vi "Main.vi"(7 "error in (no error)":errorcluster, 10 "ModuleAdmin":refnum<class "ModuleAdmin.lvclass">) -> ()   [LabVIEW 2018, in "AcPwrPlugins.lvlib"]
doc: "This VI is the critical engine of the AcPwr Plugin. It makes all the initialize, configure, and etc calls to the instrument drivers using their specifica API functions based upon the loaded configuration file."
uses:
  AcPwrPlugins.lvlib
  <userlib>/NIST/ModuleAdminLib/ModuleAdmin/ModuleAdmin.lvclass
  C:/Program Files (x86)/National Instruments/LabVIEW 2018/user.lib/NIST/ModuleAdminLib/ModuleAdminBase/ModuleAdminBase.lvclass
  AcPwrBaseClass/AcPwrBase.lvclass
  C:/Program Files (x86)/National Instruments/LabVIEW 2018/user.lib/NIST/BaseClasses/BasePlugin_class/BasePlugin.lvclass
  AcPwrShared/clStopArgument.ctl
  <userlib>/NIST/ModuleAdminLib/ModuleAdmin/ModuleAdmin.lvclass/ModuleAdmin.ctl
  <userlib>/NIST/BaseClasses/BasePlugin_class/BasePlugin.lvclass/BasePlugin.ctl
  <vilib>/Utility/error.llb/DialogType.ctl
  <userlib>/NIST/ModuleAdminLib/ModuleAdmin/Accessors/Read ShowPanel_.vi
  <userlib>/NIST/ModuleAdminLib/ModuleAdmin/Accessors/Write ShowPanel_.vi
  <userlib>/NIST/BaseClasses/BasePlugin_class/Accessors/Write PluginIniFilePath.vi
  <userlib>/NIST/BaseClasses/BasePlugin_class/Accessors/Read PluginIniFilePath.vi
  <userlib>/NIST/ModuleAdminLib/ModuleAdmin/Accessors/Read CloneRegRef.vi
  <extravilib>/ChannelInstances/Tag-bool/Read With Abort.vi
  <extravilib>/ChannelInstances/Tag-bool/Write With Abort.vi
  <extravilib>/ChannelInstances/Tag-bool/Instantiate.vi
  <extravilib>/ChannelInstances/Tag-bool/EndpointRead.vi
  <vilib>/Utility/error.llb/Error Cluster From Error Code.vi
  <extravilib>/ChannelInstances/Tag-bool/Endpoint.vi
  <vilib>/ErrorRing/Error Ring.xnode
  <userlib>/NIST/ModuleAdminLib/CloneRegistration/CloneRegistration.lvclass
  AcPwrShared/AcPwrShared.lvlib
  <userlib>/NIST/BaseClasses/Object_class/BaseObject.lvclass
  <userlib>/NIST/ModuleAdminLib/ModuleAdmin.lvlib
  <extravilib>/ChannelInstances/Tag-bool.lvlib
panel:
  out "RunTime(ms)":u32
  out "error out":errorcluster
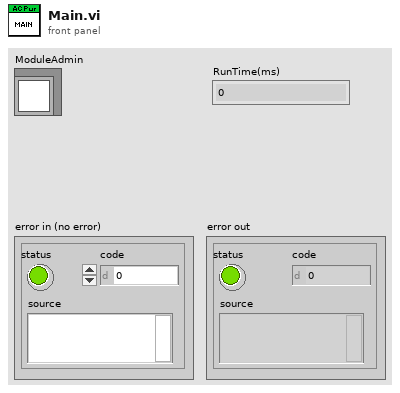
[diagram p1: front panel]
types:
  T1 = typedef "AcPwrShared.lvlib/clRequestEvents.ctl" = cluster{"StopRequest":refnum<user-event>, "PathToINI":refnum<user-event>, " LoadPlugin":refnum<user-event>, "ShowPanel":refnum<user-event>, "PrefDlg":refnum<user-event>, "InitAcPwr":refnum<user-event>, "Reset":refnum<user-event>, "Close":refnum<user-event>, "StopMeas":refnum<user-event>, "StartMeas":refnum<user-event>, "ConfigDevice":refnum<user-event>, "DeviceOn":refnum<user-event>, "DeviceOff":refnum<user-event>, "GetSettings":refnum<user-event>, "SetSettings":refnum<user-event>}
  T2 = typedef "AcPwrShared.lvlib/clBroadcastEvents.ctl" = cluster{"DidInit":refnum<user-event>, "StatusUpdate":refnum<user-event>, "ErrorReport":refnum<user-event>, "DidStop":refnum<user-event>, "PathToINI":refnum<user-event>, "Measurements":refnum<user-event>, "LoadConfigFile":refnum<user-event>, "GetSettings":refnum<user-event>, "SetSettings":refnum<user-event>, "GetType&ID":refnum<user-event>, "GotSettings":refnum<user-event>}
  T3 = typedef "AcPwrShared.lvlib/clStopArgument.ctl" = cluster{"Exit via Stop Module Req?":bool, "Wait for Module to stop?":bool, "ModuleAdmin":refnum<class "ModuleAdmin.lvclass">}
  T4 = enum32{"Invalid", "Standard", "Closed", "Hidden", "Minimized", "Maximized"}
  T5 = typedef "Tag-bool.lvlib/))Channel.ctl" = refnum<queue>
  T6 = typedef "DialogType.ctl" = u16
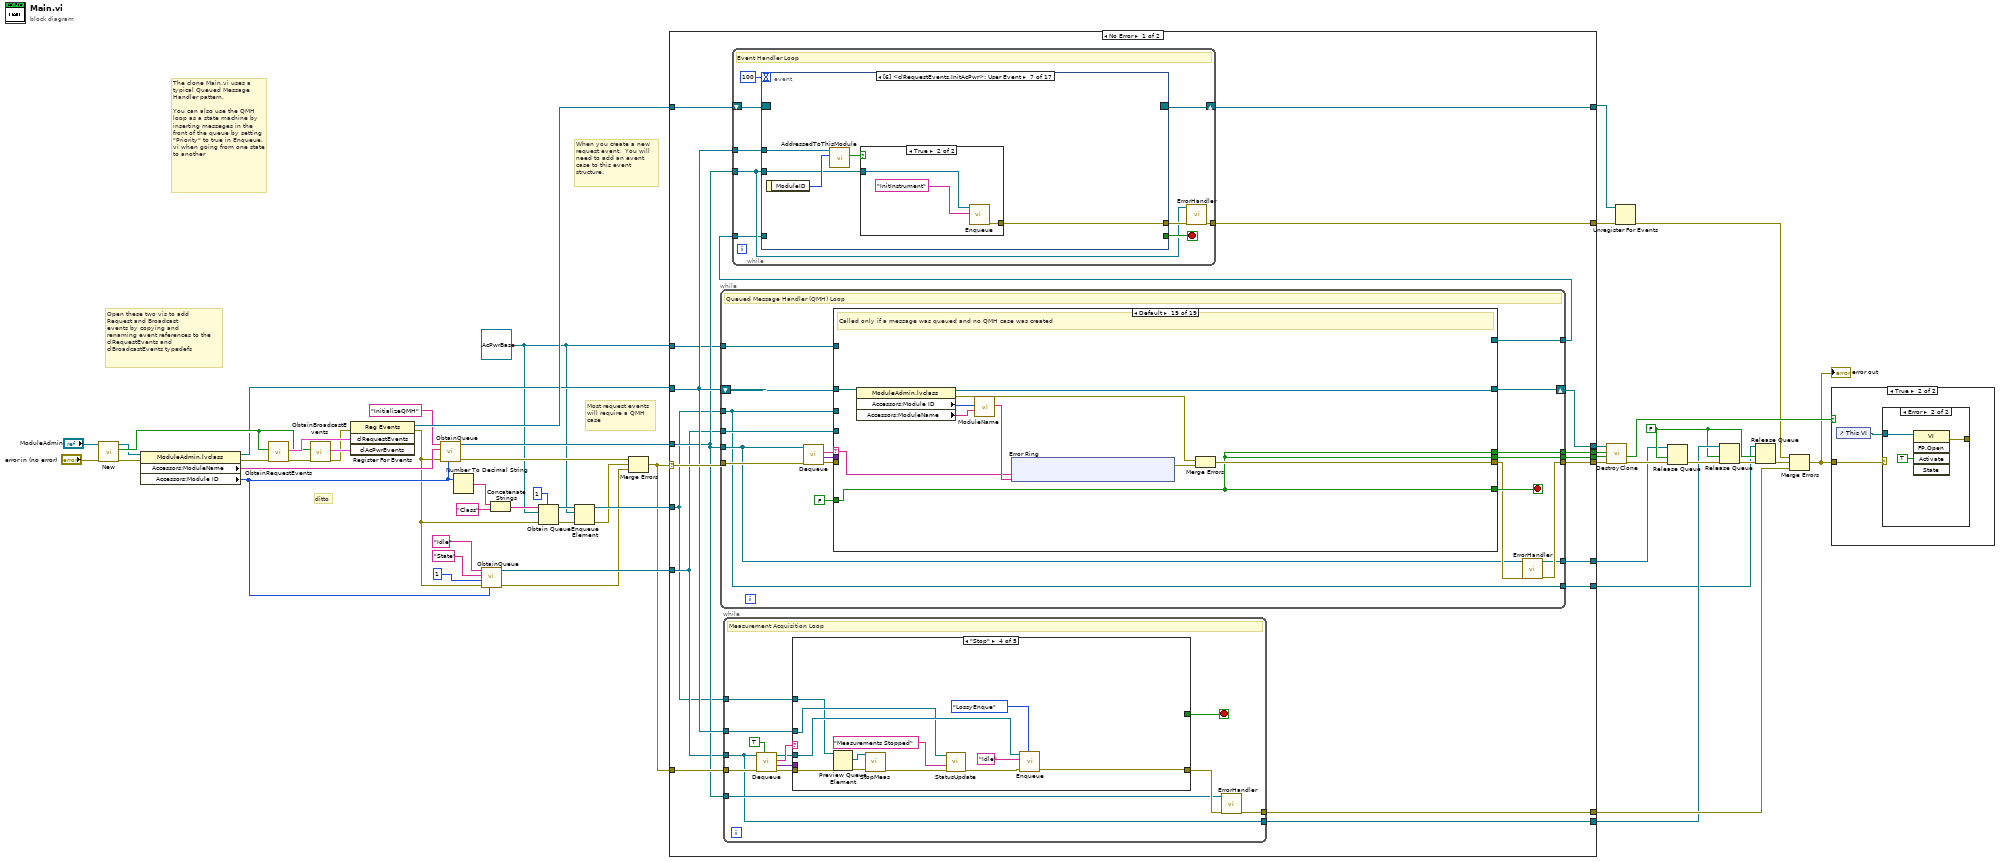
[diagram p0: block diagram]
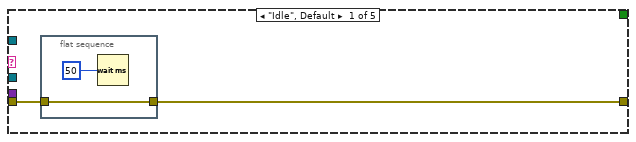
[diagram p2: hidden frame]
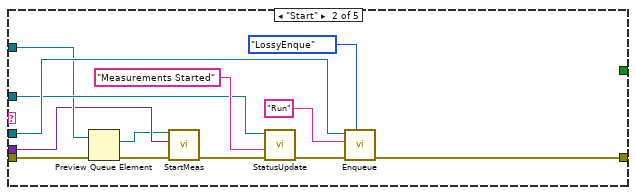
[diagram p3: hidden frame]
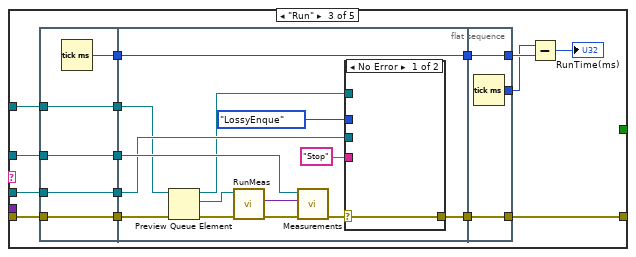
[diagram p4: hidden frame]
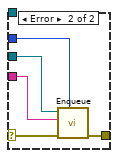
[diagram p5: hidden frame]
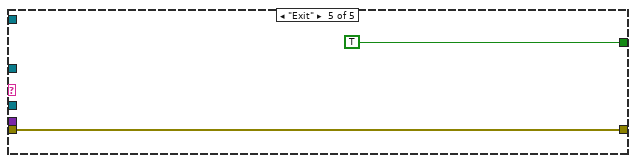
[diagram p6: hidden frame]
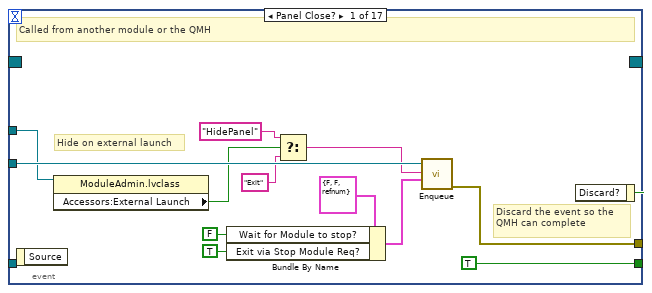
[diagram p7: hidden frame]
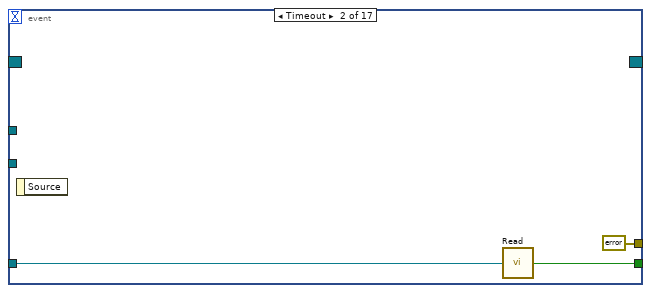
[diagram p8: hidden frame]
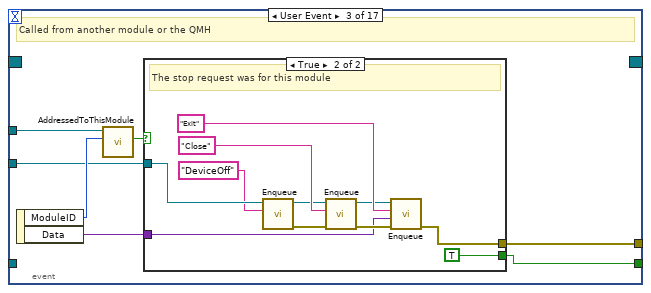
[diagram p9: hidden frame]
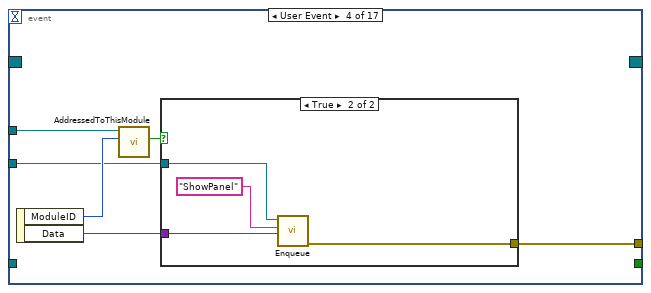
[diagram p11: hidden frame]
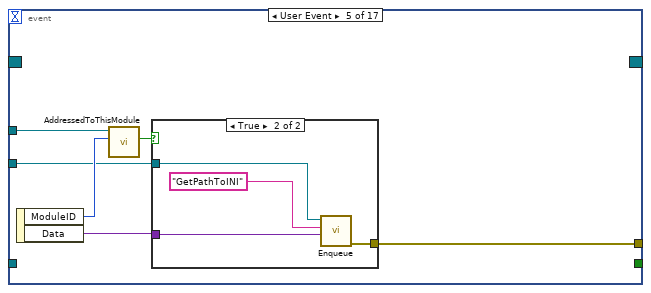
[diagram p13: hidden frame]
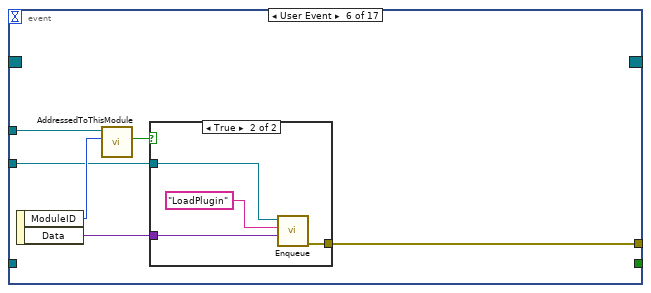
[diagram p15: hidden frame]
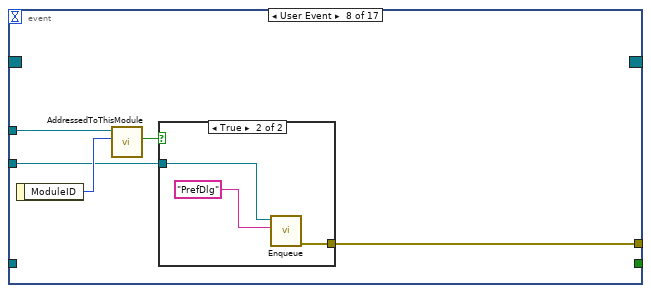
[diagram p18: hidden frame]
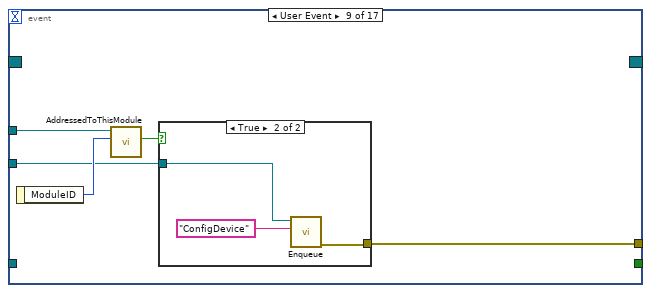
[diagram p20: hidden frame]
diagram:
  w2 = refnum<class "AcPwrBase.lvclass"> refnum ("MyPlugins.lvlib:MyPluginsBase.lvclass")
  w20 = FALSE ("force destroy? (F)")
  # "The clone Main.vi uses a typical Queued Message Handler pattern.  \n\nYou can also use the QMH loop as a state machine by inserting messeges in the front of the queue by setting \"Priority\" to true in Enqueue.vi when going from one state to another"
  # "Open these two vis to add\nRequest and Broadcast \nevents by copying and \nrenaming event references to the \nclRequestEvents and \nclBroadcastEvents typedefs"
  # "ditto"
  # "Most request events\nwill require a QMH\ncase"
  # "When you create a new request event.  You will need to add an event case to this event structure."
  n1 = call <userlib>:"New.vi"("error in (no error)"="error in (no error)", "ModuleAdmin"="ModuleAdmin") -> ("error out"=w34:errorcluster, "First?"=w47:bool, "ModuleAdmin"=w35:refnum<class "ModuleAdmin.lvclass">)  [unwired: 6 in, 1 out]
  n2 = property class="ModuleAdmin.lvclass"(reference=w35, error in=w34) -> (reference out=w31:refnum<class "ModuleAdmin.lvclass">, error out=w33:errorcluster, "Accessors:ModuleName"=w32:string, "Accessors:Module ID"=w24:i32)
  n3 = call "ObtainRequestEvents.vi"("error in (no error)"=w33, "CreateNew (F)"=w47) -> ("error out"=w46:errorcluster, "clRequestEvents"=w49:T1)  [unwired: 8 in]
  n4 = call "ObtainBroadcastEvents.vi"("error in (no error)"=w46, "CreateNew? (F)"=w47) -> ("error out"=w14:errorcluster, "clAcPwrEvents"=w45:T2)  [unwired: 8 in]
  n5 = register-events(error in=w14, w49, w45) -> (reference out=w44:refnum<event-registration>, error out=w13:errorcluster)  [unwired: 1 in]
  n6 = call "ObtainQueue.vi"("ModuleID"=w24, "error in (no error)"=w13, "ModuleName"=w32, "Initial Message"="InitializeQMH" ("ModuleName")) -> ("error out"=w9:errorcluster, "MessageQueue"=w48:refnum<queue>)  [unwired: 6 in]
  n7 = Number To Decimal String(number=w24) -> (decimal integer string=w25:string)  [unwired: 1 in]
  n8 = call "ObtainQueue.vi"("ModuleID"=w24, "error in (no error)"=w13, "max queue size (-1, unlimited)"=1, "ModuleName"="State", "Initial Message"="Idle") -> ("error out"=w7:errorcluster, "MessageQueue"=w29:refnum<queue>)  [unwired: 5 in]
  n9 = Concatenate Strings(w25, "Class" ("ModuleName")) -> (w22:string)
  n10 = Obtain Queue(max queue size (-1, unlimited)=1, name (unnamed)=w22, element data type=w2, error in (no error)=w13) -> (queue out=w16:refnum<queue>, error out=w21:errorcluster)  [unwired: 1 in, 1 out]
  n11 = Enqueue Element(queue=w16, element=w2, error in (no error)=w21) -> (queue out=w15:refnum<queue>, error out=w8:errorcluster)  [unwired: 1 in, 1 out]
  n12 = Merge Errors(w9, w8, w7) -> (w6:errorcluster)
  n13 = case shown="No Error" w6 {
    selector: w6 -> [w70 w982]
    tunnel: w48 -> [w59 w971]
    tunnel: w31 -> [w60 w980]
    tunnel: [w69 w972] -> w3
    tunnel: w44 -> [w68 w976]
    tunnel: [w67 w979] -> w4
    tunnel: [w66 _] -> w42
    tunnel: [w65 _] -> w41
    tunnel: [w64 w972] -> w39
    tunnel: [w63 w976] -> w38
    tunnel: w6 -> [w62 w975]
    tunnel: [w61 w975] -> w30
    tunnel: w29 -> [w57 w974]
    tunnel: [w58 w974] -> w27
    tunnel: w15 -> [w56 w973]
    tunnel: [w55 w973] -> w17
    tunnel: w2 -> [w53 _]
    tunnel: [w52 w971] -> w1
    frame No Error {
      n14 = while {
        tunnel: w59 -> [w343]
        tunnel: w70 -> [w352]
        tunnel: [w342] -> w69
        tunnel: [w347] -> w66
        tunnel: [w346] -> w65
        shift-right: [w344] -> w67
        shift-left: w60 -> [w348]
        tunnel: w57 -> [w341]
        tunnel: w56 -> [w340]
        tunnel: [w340] -> w55
        tunnel: [w339] -> w54
        tunnel: w53 -> [w338]
        tunnel: [w337] -> w52
        stop <- w353 stop-if-true
        # "Queued Message Handler (QMH) Loop"
        n15 = call "Dequeue.vi"("error in (no error)"=w352, "MessageQueue"=w343) -> ("error out"=w351:errorcluster, "Message Data"=w349:variant, "Message"=w350:string)  [unwired: 5 in, 2 out]
        n16 = case shown="Default" w350 {
          selector: w350 -> [_ _ _ _ _ _ _ _ _ _ _ _ _ _ _ _ _ _ w959]
          tunnel: [w354 w385 w398 w446 w458 w489 w542 w595 w608 w664 w714 w765 w773 w780 w870 w893 w917 w930 w953] -> w353
          tunnel: w348 -> [w376 w394 w403 w455 w469 w501 w554 w597 w621 w673 w722 w770 w777 w788 w885 w909 w920 w935 w962]
          tunnel: [w365 w388 w404 w456 w468 w500 w553 w603 w620 w675 w725 w771 w778 w789 w887 w910 w928 w936 w954] -> w345
          tunnel: w351 -> [w358 w397 w413 w450 w465 w499 w552 w607 w619 w671 w721 w772 w779 w784 w874 w897 w924 w933 _]
          tunnel: w349 -> [_ w396 w415 _ _ _ _ w596 w609 _ _ w766 _ _ _ _ w921 w943 _]
          tunnel: [w354 w385 w398 w446 w458 w489 w542 w595 w608 w664 w714 w765 w773 w780 w870 w893 w926 w929 w953] -> w347
          tunnel: [w354 w385 w398 w446 w458 w489 w542 w595 w608 w664 w714 w765 w773 w780 w870 w893 w925 w929 w953] -> w346
          tunnel: [w359 w393 w401 w454 w467 w496 w549 w601 w616 w672 w723 w770 w777 w787 w884 w908 w920 w934 w957] -> w344
          tunnel: w341 -> [_ _ _ _ w463 w495 w548 _ w615 w674 w724 w769 w776 w785 w872 w900 w922 _ _]
          tunnel: w340 -> [_ _ w400 w448 w462 w498 w551 w606 w618 w670 w720 _ _ w781 w875 w895 _ _ _]
          tunnel: [_ _ _ _ _ _ _ _ _ _ _ _ _ _ _ _ w916 w932 _] -> w339
          tunnel: w338 -> [_ _ w399 _ _ _ _ _ _ _ _ _ _ _ _ _ _ _ _]
          tunnel: FALSE ("Error/Exit") -> [w354 w385 w398 w446 w458 w489 w542 w595 w608 w664 w714 w765 w773 w780 w870 w893 _ w929 w953]
          frame "InitializeQMH" {
            # "After the QMH, Class, and State Queue have been created this loop enters the intialize phase."
            n17 = property class="ModuleAdmin.lvclass"(reference=w376, error in=w358) -> (reference out=w363:refnum<class "ModuleAdmin.lvclass">, error out=w373:errorcluster, "Accessors:ShowPanel_"=w362:bool, "Accessors:External Launch"=w361:bool, "Accessors:Module ID"=w356:i32, "Accessors:ModuleName"=w357:string)
            n18 = Compound Arithmetic op=OR(w362, invert w361) -> (w360:bool)
            n19 = Select(t=T4."Standard" ("Front Panel Window:State"), s=w360, f=T4."Hidden" ("Front Panel Window:State")) -> (s? t:f=w369:T4)
            n20 = invoke class="VI" method="FP.Open"(error in=w373, "State"=w369) -> (reference out=w355:refnum<vi>, error out=w372:errorcluster)  [unwired: 3 in, 3 out]
            n21 = call <userlib>:"ModuleName.vi"("Name"=w357, "ModuleID"=w356) -> ("ModuleName"=w368:string)  [unwired: 9 in]
            n22 = property class="VI"(reference=w355, error in=w372, "Front Panel.Title"=w368) -> (reference out=w375:refnum<vi>, error out=w374:errorcluster)
            n23 = invoke class="VI" method="FP.Center"(reference=w375, error in=w374) -> (error out=w364:errorcluster)  [unwired: 1 in, 2 out]
            n24 = case shown="True" w361 {
              tunnel: [w377 w383] -> w366
              tunnel: [w378 w380] -> w359
              tunnel: w364 -> [w377 w382]
              tunnel: w363 -> [w378 w379]
              frame False {
              }
              frame True {
                n25 = call <userlib>:"WaitOnModuleSync.vi"("error in (no error)"=w382, "ModuleAdmin"=w379) -> ("error out"=w384:errorcluster, "ModuleAdmin"=w381:refnum<class "ModuleAdmin.lvclass">)  [unwired: 8 in]
                n26 = call <userlib>:"WaitOnEventSync.vi"("error in (no error)"=w384, "ModuleAdmin"=w381) -> ("error out"=w383:errorcluster, "ModuleAdmin"=w380:refnum<class "ModuleAdmin.lvclass">)  [unwired: 8 in]
              }
            }
            n27 = call "DidInit.vi"("Init?"=TRUE, "error in (no error)"=w366, "ModuleAdmin"=w359) -> ("error out"=w365:errorcluster)  [unwired: 8 in]
          }
          frame "ShowPanel" {
            # "The front panel can be shown or hidden"
            n28 = Variant To Data(error in=w397, type=TRUE, Variant=w396) -> (data=w390:bool, error out=w387:errorcluster)
            n29 = property class="ModuleAdmin.lvclass"(reference=w394, error in=w387, "Accessors:ShowPanel_"=w390) -> (reference out=w393:refnum<class "ModuleAdmin.lvclass">, error out=w386:errorcluster)
            n30 = Select(t=T4."Standard" ("Front Panel Window:State"), s=w390, f=T4."Hidden" ("Front Panel Window:State")) -> (s? t:f=w389:T4)
            n31 = property class="VI"(error in=w386, "FP.State"=w389) -> (error out=w388:errorcluster)  [unwired: 1 in, 1 out]
          }
          frame "LoadPlugin" {
            # "Dynamically loads and initializes a plugin from the .ini file"
            n32 = Variant To Data(error in=w413, type=path "", Variant=w415) -> (data=w402:path, error out=w412:errorcluster)
            n33 = Current VI's Path() -> (path=w410:path)
            n34 = call <userlib>:"GetPathToClass.vi"("error in (no error)"=w412, "configuration file path"=w402) -> ("error IO"=w408:errorcluster, "PathToClass"=w411:path)  [unwired: 8 in]
            n35 = Build Path(base path=w410, name or relative path=w411) -> (appended path=w409:path)
            n36 = call <vilib>:"Check if File or Folder Exists.vi"("error in (no error)"=w408, "path"=w409) -> ("error out"=w405:errorcluster, "file or folder exists?"=w407:bool, "dup path"=w406:path)  [unwired: 7 in]
            n37 = case shown="True" w407 {
              tunnel: w406 -> [w418 w428]
              tunnel: w405 -> [_ w433]
              tunnel: [w417 w443] -> w404
              tunnel: w403 -> [w416 w439]
              tunnel: w402 -> [_ w440]
              tunnel: [w416 w438] -> w401
              tunnel: w400 -> [_ w432]
              tunnel: w399 -> [_ w427]
              frame False {
                n38 = Path To String(path=w418) -> (string=w419:string)
                n39 = xnode "Error Ring"("parameter 0"=w419) -> ("error out"=w417:errorcluster)
              }
              frame True {
                n40 = Strip Path(path=w428) -> (name=w431:string)  [unwired: 1 out]
                n41 = call-dynamic "LoadClassFromFile.vi"("error in (no error)"=w433, "class path"=w428, "reference in"=w427) -> ("error out"=w441:errorcluster, "reference out"=w442:refnum<class "AcPwrBase.lvclass">)  [unwired: 7 in]
                n42 = property class="AcPwrBase.lvclass"(reference=w442, error in=w441, "Accessors:PluginIniFilePath"=w440) -> (reference out=w437:refnum<class "AcPwrBase.lvclass">, error out=w436:errorcluster)
                n43 = call-dynamic "DefaultFromIni.vi"("error in (no error)"=w436, "AcPwrBase"=w437) -> ("error out"=w434:errorcluster, "AcPwrBase"=w435:refnum<class "AcPwrBase.lvclass">)  [unwired: 8 in]
                n44 = Lossy Enqueue Element(queue=w432, element=w435, error in (no error)=w434) -> (error out=w429:errorcluster)  [unwired: 3 out]
                n45 = Format Into String(format string="Plugin %s loaded ", error in=w429, w431) -> (resulting string=w444:string, error out=w430:errorcluster)  [unwired: 1 in]
                n46 = call "StatusUpdate.vi"("error in (no error)"=w430, "Status"=w444, "Module"=w439) -> ("error out"=w443:errorcluster, "Module"=w438:refnum<class "ModuleAdmin.lvclass">)  [unwired: 7 in]
              }
            }
          }
          frame "GetPathToINI" {
            # "Broadcast the path to the .ini file"
            n47 = Preview Queue Element(queue=w448, error in (no error)=w450) -> (element=w453:refnum<class "AcPwrBase.lvclass">, error out=w449:errorcluster)  [unwired: 1 in, 2 out]
            n48 = property class="AcPwrBase.lvclass"(reference=w453, error in=w449) -> (error out=w452:errorcluster, "Accessors:PluginIniFilePath"=w447:path)  [unwired: 1 out]
            n49 = property class="ModuleAdmin.lvclass"(reference=w455, error in=w452) -> (reference out=w454:refnum<class "ModuleAdmin.lvclass">, error out=w451:errorcluster, "Accessors:Module ID"=w457:i32)
            n50 = call "PathToINI.vi"("error in (no error)"=w451, "PathToINI"=w447, "ModuleID"=w457) -> ("error out"=w456:errorcluster)  [unwired: 8 in]
          }
          frame "InitInstrument" {
            n51 = call "Dequeue.vi"("PreviewQueue(F)"=TRUE, "error in (no error)"=w465, "MessageQueue"=w463) -> ("error out"=w464:errorcluster, "Message"=w460:string)  [unwired: 4 in, 3 out]
            n52 = Equal?(x="Run" ("y"), y=w460) -> (x = y?=w466:bool)
            n53 = case shown="False" w466 {
              tunnel: w469 -> [w481 w483]
              tunnel: [w480 w482] -> w468
              tunnel: [w478 w483] -> w467
              tunnel: w464 -> [w475 _]
              tunnel: w462 -> [w473 _]
              frame False {
                n54 = Preview Queue Element(queue=w473, error in (no error)=w475) -> (queue out=w471:refnum<queue>, element=w477:refnum<class "AcPwrBase.lvclass">, error out=w474:errorcluster)  [unwired: 1 in, 1 out]
                n55 = call-dynamic "Initialize.vi"("error in (no error)"=w474, "AcPwrBase in"=w477) -> ("error out"=w472:errorcluster, "AcPwrBase out"=w476:refnum<class "AcPwrBase.lvclass">)  [unwired: 8 in]
                n56 = Lossy Enqueue Element(queue=w471, element=w476, error in (no error)=w472) -> (error out=w470:errorcluster)  [unwired: 3 out]
                n57 = call "StatusUpdate.vi"("error in (no error)"=w470, "Status"="Device Initialized", "Module"=w481) -> ("error out"=w480:errorcluster, "Module"=w478:refnum<class "ModuleAdmin.lvclass">)  [unwired: 7 in]
              }
              frame True {
                n58 = xnode "Error Ring"() -> ("error out"=w482:errorcluster)
              }
            }
          }
          frame "ConfigDevice" {
            n59 = Preview Queue Element(queue=w498, error in (no error)=w499) -> (queue out=w497:refnum<queue>, element=w493:refnum<class "AcPwrBase.lvclass">, error out=w494:errorcluster)  [unwired: 1 in, 1 out]
            n60 = call-dynamic "ChangeWhileMeasuring.vi"("error in (no error)"=w494, "AcPwrBase in"=w493) -> ("error out"=w492:errorcluster, "OutputOrLoadValue"=w490:bool, "AcPwrBase out"=w491:refnum<class "AcPwrBase.lvclass">)  [unwired: 6 in, 1 out]
            n61 = case shown="False" w490 {
              tunnel: w501 -> [w511 w536]
              tunnel: w491 -> [w509 w518]
              tunnel: [w508 w528] -> w500
              tunnel: w492 -> [w507 w521]
              tunnel: w497 -> [w503 w525]
              tunnel: [w506 w524] -> w496
              tunnel: w495 -> [_ w520]
              frame True {
                n62 = call-dynamic "ConfigDevice.vi"("error in (no error)"=w507, "AcPwrBase in"=w509) -> ("error out"=w505:errorcluster, "AcPwrBase out"=w502:refnum<class "AcPwrBase.lvclass">)  [unwired: 8 in]
                n63 = Lossy Enqueue Element(queue=w503, element=w502, error in (no error)=w505) -> (error out=w504:errorcluster)  [unwired: 3 out]
                n64 = call "StatusUpdate.vi"("error in (no error)"=w504, "Status"="Device Configured", "Module"=w511) -> ("error out"=w508:errorcluster, "Module"=w506:refnum<class "ModuleAdmin.lvclass">)  [unwired: 7 in]
              }
              frame False {
                w533 = TRUE ("OverwriteClass? (F)")
                n65 = call "Dequeue.vi"("PreviewQueue(F)"=TRUE, "error in (no error)"=w521, "MessageQueue"=w520) -> ("error out"=w519:errorcluster, "Message"=w513:string, "MessageQueue"=w512:refnum<queue>)  [unwired: 4 in, 2 out]
                n66 = Equal?(x="Run" ("y"), y=w513) -> (x = y?=w516:bool)
                n67 = call "CheckonIdle.vi"("MessageQueue"=w512, "OverwriteClass? (F)"=w533, "error in (no error)"=w519, "ChangeOccured? (F)"=w533, "AcPwrBase in"=w518) -> ("Error Out"=w534:errorcluster, "Write?"=w530:bool, "AcPwrBase out"=w532:refnum<class "AcPwrBase.lvclass">)  [unwired: 4 in]
                n68 = call-dynamic "ConfigDevice.vi"("error in (no error)"=w534, "AcPwrBase in"=w532) -> ("error out"=w527:errorcluster, "AcPwrBase out"=w531:refnum<class "AcPwrBase.lvclass">)  [unwired: 8 in]
                n69 = case shown="True" w530 {
                  tunnel: [w537 w541] -> w526
                  tunnel: w527 -> [w537 w540]
                  tunnel: w525 -> [_ w539]
                  tunnel: w531 -> [_ w538]
                  frame False {
                  }
                  frame True {
                    n70 = Lossy Enqueue Element(queue=w539, element=w538, error in (no error)=w540) -> (error out=w541:errorcluster)  [unwired: 3 out]
                  }
                }
                n71 = call "StatusUpdate.vi"("error in (no error)"=w526, "Status"="Device Configured", "Module"=w536) -> ("error out"=w529:errorcluster, "Module"=w524:refnum<class "ModuleAdmin.lvclass">)  [unwired: 7 in]
                n72 = Select(t="Start" ("strngStateIn"), s=w516, f=w513) -> (s? t:f=w514:string)
                n73 = call "Enqueue.vi"("EnqueType (Enque)"=enum16{"LossyEnque", "EnqueAtFront", "Enque"}."LossyEnque" ("Enum"), "error in (no error)"=w529, "Message"=w514, "MessageQueue"=w512) -> ("error out"=w528:errorcluster)  [unwired: 6 in, 1 out]
              }
            }
          }
          frame "ConfigPhases" {
            # "Need to reealy look into if this case is needed"
            n74 = Preview Queue Element(queue=w551, error in (no error)=w552) -> (queue out=w550:refnum<queue>, element=w546:refnum<class "AcPwrBase.lvclass">, error out=w547:errorcluster)  [unwired: 1 in, 1 out]
            n75 = call-dynamic "ChangeWhileMeasuring.vi"("error in (no error)"=w547, "AcPwrBase in"=w546) -> ("error out"=w545:errorcluster, "OutputOrLoadValue"=w543:bool, "AcPwrBase out"=w544:refnum<class "AcPwrBase.lvclass">)  [unwired: 6 in, 1 out]
            n76 = case shown="False" w543 {
              tunnel: w554 -> [w564 w589]
              tunnel: w544 -> [w557 w575]
              tunnel: [w562 w584] -> w553
              tunnel: w545 -> [w558 w578]
              tunnel: w550 -> [w559 w582]
              tunnel: [w561 w581] -> w549
              tunnel: w548 -> [_ w577]
              frame True {
                n77 = call-dynamic "ConfigPhases.vi"("error in (no error)"=w558, "AcPwrBase in"=w557) -> ("error out"=w556:errorcluster, "AcPwrBase out"=w555:refnum<class "AcPwrBase.lvclass">)  [unwired: 8 in]
                n78 = Lossy Enqueue Element(queue=w559, element=w555, error in (no error)=w556) -> (error out=w560:errorcluster)  [unwired: 3 out]
                n79 = call "StatusUpdate.vi"("error in (no error)"=w560, "Status"="PhaseAngle Configured", "Module"=w564) -> ("error out"=w562:errorcluster, "Module"=w561:refnum<class "ModuleAdmin.lvclass">)  [unwired: 7 in]
              }
              frame False {
                w587 = TRUE ("OverwriteClass? (F)")
                n80 = call "Dequeue.vi"("PreviewQueue(F)"=TRUE, "error in (no error)"=w578, "MessageQueue"=w577) -> ("error out"=w576:errorcluster, "Message"=w570:string, "MessageQueue"=w569:refnum<queue>)  [unwired: 4 in, 2 out]
                n81 = Equal?(x="Run" ("y"), y=w570) -> (x = y?=w573:bool)
                n82 = call "CheckonIdle.vi"("MessageQueue"=w569, "OverwriteClass? (F)"=w587, "error in (no error)"=w576, "ChangeOccured? (F)"=w587, "AcPwrBase in"=w575) -> ("Error Out"=w566:errorcluster, "Write?"=w586:bool, "AcPwrBase out"=w565:refnum<class "AcPwrBase.lvclass">)  [unwired: 4 in]
                n83 = call-dynamic "ConfigPhases.vi"("error in (no error)"=w566, "AcPwrBase in"=w565) -> ("error out"=w568:errorcluster, "AcPwrBase out"=w567:refnum<class "AcPwrBase.lvclass">)  [unwired: 8 in]
                n84 = case shown="True" w586 {
                  tunnel: [w590 w594] -> w583
                  tunnel: w568 -> [w590 w593]
                  tunnel: w582 -> [_ w592]
                  tunnel: w567 -> [_ w591]
                  frame False {
                  }
                  frame True {
                    n85 = Lossy Enqueue Element(queue=w592, element=w591, error in (no error)=w593) -> (error out=w594:errorcluster)  [unwired: 3 out]
                  }
                }
                n86 = call "StatusUpdate.vi"("error in (no error)"=w583, "Status"="PhaseAngle Configured", "Module"=w589) -> ("error out"=w585:errorcluster, "Module"=w581:refnum<class "ModuleAdmin.lvclass">)  [unwired: 7 in]
                n87 = Select(t="Start" ("strngStateIn"), s=w573, f=w570) -> (s? t:f=w571:string)
                n88 = call "Enqueue.vi"("EnqueType (Enque)"=enum16{"LossyEnque", "EnqueAtFront", "Enque"}."LossyEnque" ("Enum"), "error in (no error)"=w585, "Message"=w571, "MessageQueue"=w569) -> ("error out"=w584:errorcluster)  [unwired: 6 in, 1 out]
              }
            }
          }
          frame "GetSettings" {
            n89 = Preview Queue Element(queue=w606, error in (no error)=w607) -> (element=w604:refnum<class "AcPwrBase.lvclass">, error out=w605:errorcluster)  [unwired: 1 in, 2 out]
            n90 = call-dynamic "GetSettings.vi"("error in (no error)"=w605, "SettingsToRetrieve"=w596, "AcPwrBase in"=w604) -> ("error out"=w600:errorcluster, "RetrievedSettings"=w598:variant)  [unwired: 6 in, 1 out]
            n91 = call "Settings.vi"("error in (no error)"=w600, "variant"=w598, "Module"=w597) -> ("error out"=w599:errorcluster)  [unwired: 8 in]
            n92 = call "StatusUpdate.vi"("error in (no error)"=w599, "Status"="Settings Retrieved", "Module"=w597) -> ("error out"=w603:errorcluster, "Module"=w601:refnum<class "ModuleAdmin.lvclass">)  [unwired: 7 in]
          }
          frame "SetSettings" {
            n93 = Preview Queue Element(queue=w618, error in (no error)=w619) -> (queue out=w617:refnum<queue>, element=w613:refnum<class "AcPwrBase.lvclass">, error out=w614:errorcluster)  [unwired: 1 in, 1 out]
            n94 = call-dynamic "ChangeWhileMeasuring.vi"("error in (no error)"=w614, "AcPwrBase in"=w613) -> ("error out"=w612:errorcluster, "OutputOrLoadValue"=w610:bool, "AcPwrBase out"=w611:refnum<class "AcPwrBase.lvclass">)  [unwired: 6 in, 1 out]
            n95 = case shown="False" w610 {
              tunnel: w621 -> [w632 w658]
              tunnel: w611 -> [w625 w635]
              tunnel: [w630 w653] -> w620
              tunnel: w612 -> [w626 w647]
              tunnel: w617 -> [w627 w651]
              tunnel: [w629 w650] -> w616
              tunnel: w615 -> [_ w646]
              tunnel: w609 -> [w624 w636]
              frame True {
                n96 = call-dynamic "SetSettings.vi"("error in (no error)"=w626, "Variant"=w624, "AcPwrBase in"=w625) -> ("error out"=w622:errorcluster, "AcPwrBase Out"=w623:refnum<class "AcPwrBase.lvclass">)  [unwired: 7 in]
                n97 = Lossy Enqueue Element(queue=w627, element=w623, error in (no error)=w622) -> (error out=w628:errorcluster)  [unwired: 3 out]
                n98 = call "StatusUpdate.vi"("error in (no error)"=w628, "Status"="Settings Set", "Module"=w632) -> ("error out"=w630:errorcluster, "Module"=w629:refnum<class "ModuleAdmin.lvclass">)  [unwired: 7 in]
              }
              frame False {
                w656 = TRUE ("OverwriteClass? (F)")
                n99 = call "Dequeue.vi"("PreviewQueue(F)"=TRUE, "error in (no error)"=w647, "MessageQueue"=w646) -> ("error out"=w645:errorcluster, "Message"=w640:string, "MessageQueue"=w639:refnum<queue>)  [unwired: 4 in, 2 out]
                n100 = Equal?(x="Run" ("y"), y=w640) -> (x = y?=w643:bool)
                n101 = call "CheckonIdle.vi"("MessageQueue"=w639, "OverwriteClass? (F)"=w656, "error in (no error)"=w645, "ChangeOccured? (F)"=w656, "AcPwrBase in"=w635) -> ("Error Out"=w637:errorcluster, "Write?"=w655:bool, "AcPwrBase out"=w638:refnum<class "AcPwrBase.lvclass">)  [unwired: 4 in]
                n102 = call-dynamic "SetSettings.vi"("error in (no error)"=w637, "Variant"=w636, "AcPwrBase in"=w638) -> ("error out"=w633:errorcluster, "AcPwrBase Out"=w634:refnum<class "AcPwrBase.lvclass">)  [unwired: 7 in]
                n103 = Select(t="Start" ("strngStateIn"), s=w643, f=w640) -> (s? t:f=w641:string)
                n104 = case shown="True" w655 {
                  tunnel: [w659 w663] -> w652
                  tunnel: w633 -> [w659 w662]
                  tunnel: w651 -> [_ w661]
                  tunnel: w634 -> [_ w660]
                  frame False {
                  }
                  frame True {
                    n105 = Lossy Enqueue Element(queue=w661, element=w660, error in (no error)=w662) -> (error out=w663:errorcluster)  [unwired: 3 out]
                  }
                }
                n106 = call "StatusUpdate.vi"("error in (no error)"=w652, "Status"="Settings Set", "Module"=w658) -> ("error out"=w654:errorcluster, "Module"=w650:refnum<class "ModuleAdmin.lvclass">)  [unwired: 7 in]
                n107 = call "Enqueue.vi"("EnqueType (Enque)"=enum16{"LossyEnque", "EnqueAtFront", "Enque"}."LossyEnque" ("Enum"), "error in (no error)"=w654, "Message"=w641, "MessageQueue"=w639) -> ("error out"=w653:errorcluster)  [unwired: 6 in, 1 out]
              }
            }
          }
          frame "DeviceOn" {
            # "Turns the device on."
            n108 = Preview Queue Element(queue=w670, error in (no error)=w671) -> (element=w668:refnum<class "AcPwrBase.lvclass">, error out=w669:errorcluster)  [unwired: 1 in, 2 out]
            n109 = call-dynamic "ChangeWhileMeasuring.vi"("error in (no error)"=w669, "AcPwrBase in"=w668) -> ("error out"=w667:errorcluster, "OutputOrLoadValue"=w666:bool, "AcPwrBase out"=w665:refnum<class "AcPwrBase.lvclass">)  [unwired: 6 in, 1 out]
            n110 = case shown="False" w666 {
              tunnel: [w693 w709] -> w675
              tunnel: w674 -> [w692 _]
              tunnel: w673 -> [w676 w712]
              tunnel: w670 -> [w687 _]
              tunnel: [w682 w711] -> w672
              tunnel: w667 -> [w681 w708]
              tunnel: w665 -> [_ w707]
              frame False {
                w696 = TRUE ("OverwriteClass? (F)")
                n111 = call "Dequeue.vi"("PreviewQueue(F)"=TRUE, "error in (no error)"=w681, "MessageQueue"=w692) -> ("error out"=w691:errorcluster, "Message"=w678:string, "MessageQueue"=w679:refnum<queue>)  [unwired: 4 in, 2 out]
                n112 = Preview Queue Element(queue=w687, error in (no error)=w691) -> (element=w698:refnum<class "AcPwrBase.lvclass">, error out=w690:errorcluster)  [unwired: 1 in, 2 out]
                n113 = Equal?(x="Run" ("y"), y=w678) -> (x = y?=w680:bool)
                n114 = call "CheckonIdle.vi"("MessageQueue"=w679, "OverwriteClass? (F)"=w696, "error in (no error)"=w690, "ChangeOccured? (F)"=w696, "AcPwrBase in"=w698) -> ("Error Out"=w699:errorcluster, "Write?"=w695:bool, "AcPwrBase out"=w697:refnum<class "AcPwrBase.lvclass">)  [unwired: 4 in]
                n115 = call-dynamic "DeviceOn.vi"("error in (no error)"=w699, "AcPwrBase in"=w697) -> ("error out"=w689:errorcluster, "AcPwrBase out"=w701:refnum<class "AcPwrBase.lvclass">)  [unwired: 8 in]
                n116 = case shown="True" w695 {
                  tunnel: w689 -> [w702 w706]
                  tunnel: [w702 w705] -> w688
                  tunnel: w687 -> [_ w704]
                  tunnel: w701 -> [_ w703]
                  frame False {
                  }
                  frame True {
                    n117 = Lossy Enqueue Element(queue=w704, element=w703, error in (no error)=w706) -> (error out=w705:errorcluster)  [unwired: 3 out]
                  }
                }
                n118 = call "StatusUpdate.vi"("error in (no error)"=w688, "Status"="Device On", "Module"=w676) -> ("error out"=w694:errorcluster, "Module"=w682:refnum<class "ModuleAdmin.lvclass">)  [unwired: 7 in]
                n119 = Select(t="Start" ("strngStateIn"), s=w680, f=w678) -> (s? t:f=w685:string)
                n120 = call "Enqueue.vi"("EnqueType (Enque)"=enum16{"LossyEnque", "EnqueAtFront", "Enque"}."LossyEnque" ("Enum"), "error in (no error)"=w694, "Message"=w685, "MessageQueue"=w679) -> ("error out"=w693:errorcluster)  [unwired: 6 in, 1 out]
              }
              frame True {
                n121 = call-dynamic "DeviceOn.vi"("error in (no error)"=w708, "AcPwrBase in"=w707) -> ("error out"=w710:errorcluster)  [unwired: 8 in, 1 out]
                n122 = call "StatusUpdate.vi"("error in (no error)"=w710, "Status"="Device On", "Module"=w712) -> ("error out"=w709:errorcluster, "Module"=w711:refnum<class "ModuleAdmin.lvclass">)  [unwired: 7 in]
              }
            }
          }
          frame "DeviceOff" {
            # "Turn the instruments channel off."
            n123 = Preview Queue Element(queue=w720, error in (no error)=w721) -> (element=w718:refnum<class "AcPwrBase.lvclass">, error out=w719:errorcluster)  [unwired: 1 in, 2 out]
            n124 = call-dynamic "ChangeWhileMeasuring.vi"("error in (no error)"=w719, "AcPwrBase in"=w718) -> ("error out"=w717:errorcluster, "OutputOrLoadValue"=w715:bool, "AcPwrBase out"=w716:refnum<class "AcPwrBase.lvclass">)  [unwired: 6 in, 1 out]
            n125 = case shown="False" w715 {
              tunnel: [w730 w751] -> w725
              tunnel: w724 -> [_ w749]
              tunnel: [w731 w747] -> w723
              tunnel: w722 -> [w727 w740]
              tunnel: w717 -> [w729 w734]
              tunnel: w720 -> [_ w733]
              tunnel: w716 -> [w728 _]
              frame True {
                n126 = call-dynamic "DeviceOff.vi"("error in (no error)"=w729, "AcPwrBase in"=w728) -> ("error out"=w726:errorcluster)  [unwired: 8 in, 1 out]
                n127 = call "StatusUpdate.vi"("error in (no error)"=w726, "Status"="Device Off", "Module"=w727) -> ("error out"=w730:errorcluster, "Module"=w731:refnum<class "ModuleAdmin.lvclass">)  [unwired: 7 in]
              }
              frame False {
                w756 = TRUE ("OverwriteClass? (F)")
                n128 = call "Dequeue.vi"("PreviewQueue(F)"=TRUE, "error in (no error)"=w734, "MessageQueue"=w749) -> ("error out"=w746:errorcluster, "Message"=w748:string, "MessageQueue"=w744:refnum<queue>)  [unwired: 4 in, 2 out]
                n129 = Preview Queue Element(queue=w733, error in (no error)=w746) -> (queue out=w741:refnum<queue>, element=w757:refnum<class "AcPwrBase.lvclass">, error out=w745:errorcluster)  [unwired: 1 in, 1 out]
                n130 = Equal?(x="Run" ("y"), y=w748) -> (x = y?=w750:bool)
                n131 = call "CheckonIdle.vi"("MessageQueue"=w744, "OverwriteClass? (F)"=w756, "error in (no error)"=w745, "ChangeOccured? (F)"=w756, "AcPwrBase in"=w757) -> ("Error Out"=w755:errorcluster, "Write?"=w753:bool, "AcPwrBase out"=w754:refnum<class "AcPwrBase.lvclass">)  [unwired: 4 in]
                n132 = call-dynamic "DeviceOff.vi"("error in (no error)"=w755, "AcPwrBase in"=w754) -> ("error out"=w743:errorcluster, "AcPwrBase out"=w758:refnum<class "AcPwrBase.lvclass">)  [unwired: 8 in]
                n133 = case shown="True" w753 {
                  tunnel: w743 -> [w760 w764]
                  tunnel: w758 -> [_ w763]
                  tunnel: [w760 w762] -> w742
                  tunnel: w741 -> [_ w761]
                  frame False {
                  }
                  frame True {
                    n134 = Lossy Enqueue Element(queue=w761, element=w763, error in (no error)=w764) -> (error out=w762:errorcluster)  [unwired: 3 out]
                  }
                }
                n135 = call "StatusUpdate.vi"("error in (no error)"=w742, "Status"="Device Off", "Module"=w740) -> ("error out"=w752:errorcluster, "Module"=w747:refnum<class "ModuleAdmin.lvclass">)  [unwired: 7 in]
                n136 = Select(t="Start" ("strngStateIn"), s=w750, f=w748) -> (s? t:f=w736:string)
                n137 = call "Enqueue.vi"("EnqueType (Enque)"=enum16{"LossyEnque", "EnqueAtFront", "Enque"}."LossyEnque" ("Enum"), "error in (no error)"=w752, "Message"=w736, "MessageQueue"=w744) -> ("error out"=w751:errorcluster)  [unwired: 6 in, 1 out]
              }
            }
          }
          frame "StartMeas" {
            n138 = call "Enqueue.vi"("EnqueType (Enque)"=enum16{"LossyEnque", "EnqueAtFront", "Enque"}."LossyEnque" ("Enum"), "error in (no error)"=w772, "Message Data"=w766, "Message"="Start" ("strngStateIn"), "MessageQueue"=w769) -> ("error out"=w771:errorcluster)  [unwired: 5 in, 1 out]
          }
          frame "StopMeas" {
            n139 = call "Enqueue.vi"("EnqueType (Enque)"=enum16{"LossyEnque", "EnqueAtFront", "Enque"}."LossyEnque" ("Enum"), "error in (no error)"=w779, "Message"="Stop" ("strngStateIn"), "MessageQueue"=w776) -> ("error out"=w778:errorcluster)  [unwired: 6 in, 1 out]
          }
          frame "PrefDlg" {
            # "Launch the modal Preferences dialog"
            n140 = Preview Queue Element(queue=w781, error in (no error)=w784) -> (element=w782:refnum<class "AcPwrBase.lvclass">, error out=w783:errorcluster)  [unwired: 1 in, 2 out]
            n141 = call-dynamic "PrefDialog.vi"("error in (no error)"=w783, "MyPluginsBase in"=w782) -> ("error out"=w790:errorcluster, "Save As"=w786:bool, "Changed"=w791:bool, "MyPluginsBase out"=w792:refnum<class "AcPwrBase.lvclass">)  [unwired: 6 in]
            n142 = case shown="True" w791 {
              selector: w791 -> [_ w806]
              tunnel: w792 -> [_ w801]
              tunnel: w790 -> [w797 w803]
              tunnel: [w796 w808] -> w789
              tunnel: w788 -> [w795 w809]
              tunnel: [w794 w807] -> w787
              tunnel: w786 -> [_ w802]
              tunnel: w785 -> [_ w805]
              tunnel: w781 -> [_ w804]
              frame False {
                n143 = call "StatusUpdate.vi"("error in (no error)"=w797, "Status"="Preferences Cancelled", "Module"=w795) -> ("error out"=w796:errorcluster, "Module"=w794:refnum<class "ModuleAdmin.lvclass">)  [unwired: 7 in]
              }
              frame True {
                n144 = call-dynamic "ChangeWhileMeasuring.vi"("error in (no error)"=w803, "AcPwrBase in"=w801) -> ("error out"=w799:errorcluster, "InstrumentSettings"=w798:bool, "AcPwrBase out"=w800:refnum<class "AcPwrBase.lvclass">)  [unwired: 6 in, 1 out]
                n145 = case shown="False" w798 {
                  tunnel: w809 -> [w819 w854]
                  tunnel: [w818 w853] -> w808
                  tunnel: [w810 w850] -> w807
                  tunnel: w799 -> [w814 w840]
                  tunnel: w800 -> [w811 w838]
                  tunnel: w806 -> [_ w849]
                  tunnel: w802 -> [w815 w848]
                  tunnel: w805 -> [_ w828]
                  tunnel: w804 -> [w812 w844]
                  frame True {
                    n146 = Lossy Enqueue Element(queue=w812, element=w811, error in (no error)=w814) -> (error out=w813:errorcluster)  [unwired: 3 out]
                    n147 = call "StatusUpdate.vi"("error in (no error)"=w813, "Status"="Preferences Loaded", "Module"=w819) -> ("error out"=w816:errorcluster, "Module"=w817:refnum<class "ModuleAdmin.lvclass">)  [unwired: 7 in]
                    n148 = case shown="True" w815 {
                      tunnel: [w822 w826] -> w818
                      tunnel: w817 -> [w821 w824]
                      tunnel: w816 -> [w822 w825]
                      tunnel: [w821 w823] -> w810
                      frame False {
                      }
                      frame True {
                        n149 = call "ReloadConfigurationFile.vi"("error in (no error)"=w825, "reference In"=w824) -> ("error out"=w826:errorcluster, "reference Out"=w823:refnum<class "ModuleAdmin.lvclass">)  [unwired: 8 in]
                      }
                    }
                  }
                  frame False {
                    n150 = call "Dequeue.vi"("PreviewQueue(F)"=TRUE, "error in (no error)"=w840, "MessageQueue"=w828) -> ("error out"=w839:errorcluster, "Message"=w833:string)  [unwired: 4 in, 3 out]
                    n151 = call "CheckonIdle.vi"("MessageQueue"=w828, "OverwriteClass? (F)"=w849, "error in (no error)"=w839, "ChangeOccured? (F)"=w849, "AcPwrBase in"=w838) -> ("Error Out"=w847:errorcluster, "Write?"=w845:bool, "AcPwrBase out"=w846:refnum<class "AcPwrBase.lvclass">)  [unwired: 4 in]
                    n152 = Equal?(x="Run" ("y"), y=w833) -> (x = y?=w830:bool)
                    n153 = case shown="True" w845 {
                      tunnel: w847 -> [w859 w864]
                      tunnel: [w859 w863] -> w842
                      tunnel: w844 -> [_ w862]
                      tunnel: w846 -> [w858 w861]
                      tunnel: [w858 w861] -> w829
                      tunnel: w828 -> [w857 w860]
                      tunnel: [w857 w860] -> w827
                      frame False {
                      }
                      frame True {
                        n154 = Lossy Enqueue Element(queue=w862, element=w861, error in (no error)=w864) -> (error out=w863:errorcluster)  [unwired: 3 out]
                      }
                    }
                    n155 = call-dynamic "ConnectedStatus.vi"("error in (no error)"=w842, "AcPwrBase in"=w829) -> ("error out"=w843:errorcluster, "Any Connections"=w832:bool)  [unwired: 7 in, 1 out]
                    n156 = And(x=w832, y=w830) -> (x .and. y?=w831:bool)
                    n157 = Select(t="Start" ("strngStateIn"), s=w831, f=w833) -> (s? t:f=w834:string)
                    n158 = call "Enqueue.vi"("EnqueType (Enque)"=enum16{"LossyEnque", "EnqueAtFront", "Enque"}."LossyEnque" ("Enum"), "error in (no error)"=w843, "Message"=w834, "MessageQueue"=w827) -> ("error out"=w855:errorcluster)  [unwired: 6 in, 1 out]
                    n159 = call "StatusUpdate.vi"("error in (no error)"=w855, "Status"="Preferences Loaded", "Module"=w854) -> ("error out"=w851:errorcluster, "Module"=w852:refnum<class "ModuleAdmin.lvclass">)  [unwired: 7 in]
                    n160 = case shown="True" w848 {
                      tunnel: [w865 w869] -> w853
                      tunnel: w852 -> [w866 w867]
                      tunnel: w851 -> [w865 w868]
                      tunnel: [w866 w867] -> w850
                      frame False {
                      }
                      frame True {
                        n161 = call "ReloadConfigurationFile.vi"("error in (no error)"=w868, "reference In"=w867) -> ("error out"=w869:errorcluster)  [unwired: 8 in, 1 out]
                      }
                    }
                  }
                }
              }
            }
          }
          frame "Reset" {
            w881 = TRUE ("btnSet")
            n162 = Preview Queue Element(queue=w875, error in (no error)=w874) -> (queue out=w871:refnum<queue>, element=w882:refnum<class "AcPwrBase.lvclass">, error out=w873:errorcluster)  [unwired: 1 in, 1 out]
            n163 = call "CheckonIdle.vi"("MessageQueue"=w872, "OverwriteClass? (F)"=w881, "error in (no error)"=w873, "ChangeOccured? (F)"=w881, "AcPwrBase in"=w882) -> ("Error Out"=w880:errorcluster, "Write?"=w878:bool, "AcPwrBase out"=w879:refnum<class "AcPwrBase.lvclass">)  [unwired: 4 in]
            n164 = call-dynamic "Reset.vi"("error in (no error)"=w880, "AcPwrBase in"=w879) -> ("error out"=w877:errorcluster, "AcPwrBase out"=w883:refnum<class "AcPwrBase.lvclass">)  [unwired: 8 in]
            n165 = case shown="True" w878 {
              tunnel: w877 -> [w888 w892]
              tunnel: [w888 w891] -> w876
              tunnel: w883 -> [_ w890]
              tunnel: w871 -> [_ w889]
              frame False {
              }
              frame True {
                n166 = Lossy Enqueue Element(queue=w889, element=w890, error in (no error)=w892) -> (error out=w891:errorcluster)  [unwired: 3 out]
              }
            }
            n167 = call "StatusUpdate.vi"("error in (no error)"=w876, "Status"="Device Reset", "Module"=w885) -> ("error out"=w887:errorcluster, "Module"=w884:refnum<class "ModuleAdmin.lvclass">)  [unwired: 7 in]
          }
          frame "Close" {
            w901 = TRUE ("btnSet")
            n168 = Preview Queue Element(queue=w895, error in (no error)=w897) -> (queue out=w894:refnum<queue>, element=w902:refnum<class "AcPwrBase.lvclass">, error out=w896:errorcluster)  [unwired: 1 in, 1 out]
            n169 = call "CheckonIdle.vi"("MessageQueue"=w900, "OverwriteClass? (F)"=w901, "error in (no error)"=w896, "ChangeOccured? (F)"=w901, "AcPwrBase in"=w902) -> ("Error Out"=w905:errorcluster, "Write?"=w903:bool, "AcPwrBase out"=w904:refnum<class "AcPwrBase.lvclass">)  [unwired: 4 in]
            n170 = call-dynamic "Close.vi"("error in (no error)"=w905, "AcPwrBase in"=w904) -> ("error out"=w899:errorcluster, "AcPwrBase out"=w906:refnum<class "AcPwrBase.lvclass">)  [unwired: 8 in]
            n171 = case shown="True" w903 {
              tunnel: w899 -> [w911 w915]
              tunnel: [w911 w914] -> w898
              tunnel: w906 -> [_ w913]
              tunnel: w894 -> [_ w912]
              frame False {
              }
              frame True {
                n172 = Lossy Enqueue Element(queue=w912, element=w913, error in (no error)=w915) -> (error out=w914:errorcluster)  [unwired: 3 out]
              }
            }
            n173 = call "StatusUpdate.vi"("error in (no error)"=w898, "Status"="Device Closed", "Module"=w909) -> ("error out"=w910:errorcluster, "Module"=w908:refnum<class "ModuleAdmin.lvclass">)  [unwired: 7 in]
          }
          frame "Exit" {
            w917 = TRUE ("Error/Exit")
            # "Called by the StopRequest event handler case"
            n174 = control-ref of="This VI"() -> (w927:refnum<vi>)
            n175 = call "Enqueue.vi"("EnqueType (Enque)"=enum16{"LossyEnque", "EnqueAtFront", "Enque"}."LossyEnque" ("Enum"), "error in (no error)"=w924, "Message"="Exit" ("strngStateIn"), "MessageQueue"=w922) -> ("error out"=w923:errorcluster)  [unwired: 6 in, 1 out]
            n176 = call "HandleExit.vi"("error in (no error)"=w923, "VI Refnum"=w927, "StopArgument"=w921, "ModuleAdmin"=w920) -> ("error out"=w928:errorcluster, "Exit via Stop Module Req?"=w925:bool, "WaitForStop?"=w926:bool)  [unwired: 5 in]
            n177 = call <extravilib>:"Write.vi"("element"=w917) -> ("channel"=w916:T5)  [unwired: 1 out]
          }
          frame "Error" {
            # "Handle any errors"
            n178 = property class="ModuleAdmin.lvclass"(reference=w935, error in=w933) -> (reference out=w934:refnum<class "ModuleAdmin.lvclass">, error out=w931:errorcluster, "Accessors:External Launch"=w939:bool, "Accessors:Module ID"=w937:i32)
            n179 = Variant To Data(error in=w931, type=errorcluster {"status"=FALSE, "code"=0, "source"=""} ("error constant"), Variant=w943) -> (data=w938:errorcluster, error out=w941:errorcluster)
            n180 = call "ReportError.vi"("error in (no error)"=w941, "ErrorReported"=w938, "ModuleID"=w937) -> ("error out"=w940:errorcluster)  [unwired: 8 in]
            n181 = case shown="False" w939 {
              tunnel: w940 -> [w948 w952]
              tunnel: w938 -> [w950 _]
              tunnel: [w948 w952] -> w936
              tunnel: [w944 w951] -> w930
              frame False {
                w949 = T6 0 items=["no dialog", "OK message", "continue or stop message", "OK message + warnings", "continue/stop + warnings"] ("type of dialog (OK msg:1)")
                # "Stand alone: now, force an exit"
                n182 = call <vilib>:"Simple Error Handler.vi"("type of dialog (OK msg:1)"=w949, "error in (no error)"=w950) -> ("message"=w945:string)  [unwired: 3 in, 4 out]
                n183 = Two Button Dialog(message=w945, 1:"Continue" ("F button name (\"Cancel\")"), 2:"Exit" ("T button name (\"OK\")")) -> (T button?=w944:bool)
              }
              frame True {
                w951 = FALSE  # Error/Exit
                # "Externally launched modules only broadcast the error msg"
              }
            }
            n184 = call <extravilib>:"Write.vi"("element"=w930) -> ("channel"=w932:T5)  [unwired: 1 out]
          }
          frame Default {
            # "Called only if a message was queued and no QMH case was created"
            n185 = property class="ModuleAdmin.lvclass"(reference=w962) -> (reference out=w957:refnum<class "ModuleAdmin.lvclass">, error out=w956:errorcluster, "Accessors:Module ID"=w961:i32, "Accessors:ModuleName"=w958:string)  [unwired: 1 in]
            n186 = call <userlib>:"ModuleName.vi"("Name"=w958, "ModuleID"=w961) -> ("ModuleName"=w960:string)  [unwired: 9 in]
            n187 = xnode "Error Ring"("parameter 0"=w959, "parameter 1"=w960) -> ("error out"=w955:errorcluster)
            n188 = Merge Errors(w956, w955) -> (w954:errorcluster)
          }
        }
        n189 = call "ErrorHandler.vi"("error in (no error)"=w345, "MessageQueue"=w343) -> ("error out"=w342:errorcluster, "MessageQueue"=w337:refnum<queue>)  [unwired: 8 in]
      }
      n190 = while {
        tunnel: w62 -> [w79]
        tunnel: [w76] -> w61
        tunnel: w60 -> [w82]
        tunnel: w59 -> [w80]
        tunnel: w57 -> [w75]
        tunnel: [w75] -> w58
        tunnel: w56 -> [w72]
        stop <- w83 stop-if-true
        # "Measurement Acquisition Loop"
        n191 = call "Dequeue.vi"("PreviewQueue(F)"=TRUE, "error in (no error)"=w79, "MessageQueue"=w75) -> ("error out"=w78:errorcluster, "Message Data"=w71:variant, "Message"=w77:string, "MessageQueue"=w74:refnum<queue>)  [unwired: 4 in, 1 out]
        n192 = case shown="\"Stop\"" w77 {
          tunnel: [_ _ _ _ TRUE] -> w83
          tunnel: w78 -> [w84 w90 w112 w149 w156]
          tunnel: [w85 w97 w114 w151 w156] -> w81
          tunnel: w82 -> [_ w94 w115 w147 _]
          tunnel: w74 -> [_ w96 w113 w150 _]
          tunnel: w72 -> [_ w93 w111 w146 _]
          tunnel: w71 -> [_ w89 _ _ _]
          frame "Idle", Default {
            n193 = flat-sequence {
              tunnel: [w86] -> w85
              tunnel: w84 -> [w86]
              frame #0 {
                n194 = Wait (ms)(milliseconds to wait=u32 50) -> ()  [unwired: 1 out]
              }
            }
          }
          frame "Start" {
            n195 = Preview Queue Element(queue=w93, error in (no error)=w90) -> (element=w88:refnum<class "AcPwrBase.lvclass">, error out=w95:errorcluster)  [unwired: 1 in, 2 out]
            n196 = call-dynamic "StartMeas.vi"("error in (no error)"=w95, "Variant"=w89, "AcPwrBase in"=w88) -> ("error out"=w99:errorcluster)  [unwired: 7 in, 1 out]
            n197 = call "StatusUpdate.vi"("error in (no error)"=w99, "Status"="Measurements Started", "Module"=w94) -> ("error out"=w98:errorcluster)  [unwired: 7 in, 1 out]
            n198 = call "Enqueue.vi"("EnqueType (Enque)"=enum16{"LossyEnque", "EnqueAtFront", "Enque"}."LossyEnque" ("Enum"), "error in (no error)"=w98, "Message"="Run" ("strngStateIn"), "MessageQueue"=w96) -> ("error out"=w97:errorcluster)  [unwired: 6 in, 1 out]
          }
          frame "Run" {
            n199 = flat-sequence {
              tunnel: w111 -> [w117]
              tunnel: w112 -> [w118]
              tunnel: w113 -> [w119]
              tunnel: w115 -> [w120]
              tunnel: [w120] -> w109
              tunnel: [w119] -> w108
              tunnel: [w118] -> w107
              tunnel: [w117] -> w106
              tunnel: [w116] -> w104
              tunnel: [w131] -> w110
              tunnel: w109 -> [w133]
              tunnel: w108 -> [w128]
              tunnel: w107 -> [w126]
              tunnel: w106 -> [w125]
              tunnel: [w121] -> w105
              tunnel: w104 -> [w121]
              tunnel: [w143] -> w114
              tunnel: w110 -> [w143]
              tunnel: w105 -> [w142]
              tunnel: [w142] -> w103
              tunnel: [w141] -> w102
              frame #0 {
                n200 = Tick Count (ms)() -> (millisecond timer value=w116:u32)
              }
              frame #1 {
                n201 = Preview Queue Element(queue=w125, error in (no error)=w126) -> (queue out=w122:refnum<queue>, element=w134:refnum<class "AcPwrBase.lvclass">, error out=w127:errorcluster)  [unwired: 1 in, 1 out]
                n202 = call-dynamic "RunMeas.vi"("error in (no error)"=w127, "AcPwrBase in"=w134) -> ("error out"=w130:errorcluster, "variant"=w129:variant)  [unwired: 7 in, 1 out]
                n203 = call "Measurements.vi"("error in (no error)"=w130, "Variant"=w129, "Module"=w133) -> ("error out"=w132:errorcluster)  [unwired: 8 in]
                n204 = case shown="No Error" w132 {
                  selector: w132 -> [w135 w136]
                  tunnel: [w135 w140] -> w131
                  tunnel: w128 -> [_ w139]
                  tunnel: enum16{"LossyEnque", "EnqueAtFront", "Enque"}."LossyEnque" ("Enum") -> [_ w137]
                  tunnel: "Stop" ("strngStateIn") -> [_ w138]
                  tunnel: w122 -> [_ _]
                  frame No Error {
                  }
                  frame Error {
                    n205 = call "Enqueue.vi"("EnqueType (Enque)"=w137, "error in (no error)"=w136, "Message"=w138, "MessageQueue"=w139) -> ("error out"=w140:errorcluster)  [unwired: 6 in, 1 out]
                  }
                }
              }
              frame #2 {
                n206 = Tick Count (ms)() -> (millisecond timer value=w141:u32)
              }
            }
            n207 = Subtract(x=w102, y=w103) -> (x-y=→"RunTime(ms)":u32)
          }
          frame "Stop" {
            n208 = Preview Queue Element(queue=w146, error in (no error)=w149) -> (element=w155:refnum<class "AcPwrBase.lvclass">, error out=w148:errorcluster)  [unwired: 1 in, 2 out]
            n209 = call-dynamic "StopMeas.vi"("error in (no error)"=w148, "AcPwrBase in"=w155) -> ("error out"=w153:errorcluster)  [unwired: 8 in, 1 out]
            n210 = call "StatusUpdate.vi"("error in (no error)"=w153, "Status"="Measurements Stopped", "Module"=w147) -> ("error out"=w152:errorcluster)  [unwired: 7 in, 1 out]
            n211 = call "Enqueue.vi"("EnqueType (Enque)"=enum16{"LossyEnque", "EnqueAtFront", "Enque"}."LossyEnque" ("Enum"), "error in (no error)"=w152, "Message"="Idle" ("strngStateIn"), "MessageQueue"=w150) -> ("error out"=w151:errorcluster)  [unwired: 6 in, 1 out]
          }
          frame "Exit" {
          }
        }
        n212 = call "ErrorHandler.vi"("error in (no error)"=w81, "MessageQueue"=w80) -> ("error out"=w76:errorcluster)  [unwired: 8 in, 1 out]
      }
      n213 = while {
        tunnel: w59 -> [w160]
        shift-right: [w164] -> w63
        shift-left: w68 -> [w165]
        tunnel: w60 -> [w163]
        tunnel: [w161] -> w64
        tunnel: w54 -> [w158]
        stop <- w166 stop-if-true
        # "Event Handler Loop"
        n214 = event shown="[6] <clRequestEvents.InitAcPwr>: User Event" {
          selector: w165 -> [_ _ _ _ _ _ _ _ _ _ _ _ _ _ _ _ _]
          dyn-events: [_ _ _ _ _ _ _ _ _ _ _ _ _ _ _ _ _] -> w164
          timeout: 100 -> [_ _ _ _ _ _ _ _ _ _ _ _ _ _ _ _ _]
          tunnel: w160 -> [w179 _ w186 w203 w214 w223 w233 w240 w248 w257 w267 w277 w286 w295 w304 w312 w323]
          tunnel: [TRUE w180 w185 _ _ _ _ _ _ _ _ _ _ _ _ _ _] -> w166
          tunnel: w163 -> [w173 _ w189 w207 w213 w227 w236 w244 w252 w261 w271 w280 w289 w297 w306 w316 w322]
          tunnel: [w177 errorcluster {"status"=FALSE, "code"=0, "source"=""} ("error out") w184 w204 w212 w224 w232 w241 w249 w258 w268 w276 w284 w296 w305 w313 w324] -> w162
          tunnel: w158 -> [_ w181 _ _ _ _ _ _ _ _ _ _ _ _ _ _ _]
          event Panel Close? {
            # "Hide on external launch"
            # "Discard the event so the QMH can complete"
            # "Called from another module or the QMH"
            n215 = event-data() -> ()  [unwired: 1 in, 1 out]
            n216 = property class="ModuleAdmin.lvclass"(reference=w173) -> ("Accessors:External Launch"=w168:bool)  [unwired: 1 in, 2 out]
            n217 = Bundle By Name(cluster=T3 {"Exit via Stop Module Req?"=FALSE, "Wait for Module to stop?"=FALSE, "ModuleAdmin"=refnum} ("Stop Argument"), "Wait for Module to stop?"=FALSE, "Exit via Stop Module Req?"=TRUE) -> (w174:T3)
            n218 = Select(t="HidePanel", s=w168, f="Exit" ("Message")) -> (s? t:f=w170:string)
            n219 = call "Enqueue.vi"("Message Data"=w174, "Message"=w170, "MessageQueue"=w179) -> ("error out"=w177:errorcluster)  [unwired: 7 in, 1 out]
            n220 = event-data("Discard?"=TRUE) -> ()  [unwired: 1 in, 1 out]
          }
          event Timeout {
            n221 = event-data() -> ()  [unwired: 1 in, 1 out]
            n222 = call <extravilib>:"Read.vi"("channel"=w181) -> ("element"=w180:bool)  [unwired: 1 in, 1 out]
          }
          event User Event {
            # "Called from another module or the QMH"
            n223 = event-data() -> ("ModuleID"=w187:i32, "Data"=w183:variant)  [unwired: 1 in]
            n224 = call <userlib>:"AddressedToThisModule.vi"("ModuleID"=w187, "ModuleAdmin"=w189) -> ("AddressedToThisInstance?"=w188:bool)  [unwired: 8 in, 1 out]
            n225 = case shown="True" w188 {
              tunnel: w186 -> [_ w193]
              tunnel: [FALSE TRUE] -> w185
              tunnel: [_ w197] -> w184
              tunnel: w183 -> [_ w191]
              frame False {
                # "The stop request was for a different module"
              }
              frame True {
                # "The stop request was for this module"
                n226 = call "Enqueue.vi"("Message"="DeviceOff", "MessageQueue"=w193) -> ("error out"=w195:errorcluster, "MessageQueue"=w194:refnum<queue>)  [unwired: 8 in]
                n227 = call "Enqueue.vi"("error in (no error)"=w195, "Message"="Close", "MessageQueue"=w194) -> ("error out"=w198:errorcluster, "MessageQueue"=w196:refnum<queue>)  [unwired: 7 in]
                n228 = call "Enqueue.vi"("error in (no error)"=w198, "Message Data"=w191, "Message"="Exit", "MessageQueue"=w196) -> ("error out"=w197:errorcluster)  [unwired: 6 in, 1 out]
              }
            }
          }
          event User Event {
            n229 = event-data() -> ("ModuleID"=w206:i32, "Data"=w202:variant)  [unwired: 1 in]
            n230 = call <userlib>:"AddressedToThisModule.vi"("ModuleID"=w206, "ModuleAdmin"=w207) -> ("AddressedToThisInstance?"=w205:bool)  [unwired: 8 in, 1 out]
            n231 = case shown="True" w205 {
              tunnel: [_ w208] -> w204
              tunnel: w203 -> [_ w211]
              tunnel: w202 -> [_ w209]
              frame False {
              }
              frame True {
                n232 = call "Enqueue.vi"("Message Data"=w209, "Message"="ShowPanel", "MessageQueue"=w211) -> ("error out"=w208:errorcluster)  [unwired: 7 in, 1 out]
              }
            }
          }
          event User Event {
            n233 = event-data() -> ("ModuleID"=w215:i32, "Data"=w216:variant)  [unwired: 1 in]
            n234 = call <userlib>:"AddressedToThisModule.vi"("ModuleID"=w215, "ModuleAdmin"=w213) -> ("AddressedToThisInstance?"=w217:bool)  [unwired: 8 in, 1 out]
            n235 = case shown="True" w217 {
              tunnel: w214 -> [_ w221]
              tunnel: [_ w220] -> w212
              tunnel: w216 -> [_ w218]
              frame False {
                (unwired) FALSE
                # "The stop request was for a different module"
              }
              frame True {
                # "The stop request was for this module"
                n236 = call "Enqueue.vi"("Message Data"=w218, "Message"="GetPathToINI", "MessageQueue"=w221) -> ("error out"=w220:errorcluster)  [unwired: 7 in, 1 out]
              }
            }
          }
          event User Event {
            n237 = event-data() -> ("ModuleID"=w226:i32, "Data"=w222:variant)  [unwired: 1 in]
            n238 = call <userlib>:"AddressedToThisModule.vi"("ModuleID"=w226, "ModuleAdmin"=w227) -> ("AddressedToThisInstance?"=w225:bool)  [unwired: 8 in, 1 out]
            n239 = case shown="True" w225 {
              tunnel: [_ w228] -> w224
              tunnel: w223 -> [_ w231]
              tunnel: w222 -> [_ w229]
              frame False {
              }
              frame True {
                n240 = call "Enqueue.vi"("Message Data"=w229, "Message"="LoadPlugin", "MessageQueue"=w231) -> ("error out"=w228:errorcluster)  [unwired: 7 in, 1 out]
              }
            }
          }
          event User Event {
            n241 = event-data() -> ("ModuleID"=w235:i32)  [unwired: 1 in]
            n242 = call <userlib>:"AddressedToThisModule.vi"("ModuleID"=w235, "ModuleAdmin"=w236) -> ("AddressedToThisInstance?"=w234:bool)  [unwired: 8 in, 1 out]
            n243 = case shown="True" w234 {
              tunnel: w233 -> [_ w238]
              tunnel: [_ w237] -> w232
              frame False {
              }
              frame True {
                n244 = call "Enqueue.vi"("Message"="InitInstrument", "MessageQueue"=w238) -> ("error out"=w237:errorcluster)  [unwired: 8 in, 1 out]
              }
            }
          }
          event User Event {
            n245 = event-data() -> ("ModuleID"=w243:i32)  [unwired: 1 in]
            n246 = call <userlib>:"AddressedToThisModule.vi"("ModuleID"=w243, "ModuleAdmin"=w244) -> ("AddressedToThisInstance?"=w242:bool)  [unwired: 8 in, 1 out]
            n247 = case shown="True" w242 {
              tunnel: [_ w245] -> w241
              tunnel: w240 -> [_ w247]
              frame False {
              }
              frame True {
                n248 = call "Enqueue.vi"("Message"="PrefDlg", "MessageQueue"=w247) -> ("error out"=w245:errorcluster)  [unwired: 8 in, 1 out]
              }
            }
          }
          event User Event {
            n249 = event-data() -> ("ModuleID"=w251:i32)  [unwired: 1 in]
            n250 = call <userlib>:"AddressedToThisModule.vi"("ModuleID"=w251, "ModuleAdmin"=w252) -> ("AddressedToThisInstance?"=w250:bool)  [unwired: 8 in, 1 out]
            n251 = case shown="True" w250 {
              tunnel: [_ w255] -> w249
              tunnel: w248 -> [_ w253]
              frame False {
              }
              frame True {
                n252 = call "Enqueue.vi"("Message"="ConfigDevice", "MessageQueue"=w253) -> ("error out"=w255:errorcluster)  [unwired: 8 in, 1 out]
              }
            }
          }
          event User Event {
            n253 = event-data() -> ("ModuleID"=w260:i32, "Data"=w256:variant)  [unwired: 1 in]
            n254 = call <userlib>:"AddressedToThisModule.vi"("ModuleID"=w260, "ModuleAdmin"=w261) -> ("AddressedToThisInstance?"=w259:bool)  [unwired: 8 in, 1 out]
            n255 = case shown="True" w259 {
              tunnel: [_ w263] -> w258
              tunnel: w257 -> [_ w264]
              tunnel: w256 -> [_ w262]
              frame False {
              }
              frame True {
                n256 = call "Enqueue.vi"("Message Data"=w262, "Message"="GetSettings", "MessageQueue"=w264) -> ("error out"=w263:errorcluster)  [unwired: 7 in, 1 out]
              }
            }
          }
          event User Event {
            n257 = event-data() -> ("ModuleID"=w270:i32, "Data"=w266:variant)  [unwired: 1 in]
            n258 = call <userlib>:"AddressedToThisModule.vi"("ModuleID"=w270, "ModuleAdmin"=w271) -> ("AddressedToThisInstance?"=w269:bool)  [unwired: 8 in, 1 out]
            n259 = case shown="True" w269 {
              tunnel: [_ w272] -> w268
              tunnel: w267 -> [_ w274]
              tunnel: w266 -> [_ w273]
              frame False {
              }
              frame True {
                n260 = call "Enqueue.vi"("Message Data"=w273, "Message"="SetSettings", "MessageQueue"=w274) -> ("error out"=w272:errorcluster)  [unwired: 7 in, 1 out]
              }
            }
          }
          event User Event {
            n261 = event-data() -> ("ModuleID"=w279:i32)  [unwired: 1 in]
            n262 = call <userlib>:"AddressedToThisModule.vi"("ModuleID"=w279, "ModuleAdmin"=w280) -> ("AddressedToThisInstance?"=w278:bool)  [unwired: 8 in, 1 out]
            n263 = case shown="True" w278 {
              tunnel: w277 -> [_ w282]
              tunnel: [_ w281] -> w276
              frame False {
              }
              frame True {
                n264 = call "Enqueue.vi"("Message"="DeviceOn", "MessageQueue"=w282) -> ("error out"=w281:errorcluster)  [unwired: 8 in, 1 out]
              }
            }
          }
          event User Event {
            n265 = event-data() -> ("ModuleID"=w288:i32, "Data"=w285:variant)  [unwired: 1 in]
            n266 = call <userlib>:"AddressedToThisModule.vi"("ModuleID"=w288, "ModuleAdmin"=w289) -> ("AddressedToThisInstance?"=w287:bool)  [unwired: 8 in, 1 out]
            n267 = case shown="True" w287 {
              tunnel: w286 -> [_ w292]
              tunnel: w285 -> [_ w291]
              tunnel: [_ w290] -> w284
              frame False {
              }
              frame True {
                n268 = call "Enqueue.vi"("Message Data"=w291, "Message"="DeviceOff", "MessageQueue"=w292) -> ("error out"=w290:errorcluster)  [unwired: 7 in, 1 out]
              }
            }
          }
          event User Event {
            n269 = event-data() -> ("ModuleID"=w299:i32, "Data"=w294:variant)  [unwired: 1 in]
            n270 = call <userlib>:"AddressedToThisModule.vi"("ModuleID"=w299, "ModuleAdmin"=w297) -> ("AddressedToThisInstance?"=w298:bool)  [unwired: 8 in, 1 out]
            n271 = case shown="True" w298 {
              tunnel: [_ w302] -> w296
              tunnel: w295 -> [_ w301]
              tunnel: w294 -> [_ w300]
              frame False {
              }
              frame True {
                n272 = call "Enqueue.vi"("Message Data"=w300, "Message"="StartMeas", "MessageQueue"=w301) -> ("error out"=w302:errorcluster)  [unwired: 7 in, 1 out]
              }
            }
          }
          event User Event {
            n273 = event-data() -> ("ModuleID"=w307:i32)  [unwired: 1 in]
            n274 = call <userlib>:"AddressedToThisModule.vi"("ModuleID"=w307, "ModuleAdmin"=w306) -> ("AddressedToThisInstance?"=w308:bool)  [unwired: 8 in, 1 out]
            n275 = case shown="True" w308 {
              tunnel: [_ w309] -> w305
              tunnel: w304 -> [_ w310]
              frame False {
              }
              frame True {
                n276 = call "Enqueue.vi"("Message"="StopMeas", "MessageQueue"=w310) -> ("error out"=w309:errorcluster)  [unwired: 8 in, 1 out]
              }
            }
          }
          event User Event {
            n277 = event-data() -> ("ModuleID"=w315:i32)  [unwired: 1 in]
            n278 = call <userlib>:"AddressedToThisModule.vi"("ModuleID"=w315, "ModuleAdmin"=w316) -> ("AddressedToThisInstance?"=w314:bool)  [unwired: 8 in, 1 out]
            n279 = case shown="True" w314 {
              tunnel: [_ w319] -> w313
              tunnel: w312 -> [_ w317]
              frame False {
              }
              frame True {
                n280 = call "Enqueue.vi"("Message"="Reset", "MessageQueue"=w317) -> ("error out"=w319:errorcluster)  [unwired: 8 in, 1 out]
              }
            }
          }
          event User Event {
            n281 = event-data() -> ("ModuleID"=w321:i32)  [unwired: 1 in]
            n282 = call <userlib>:"AddressedToThisModule.vi"("ModuleID"=w321, "ModuleAdmin"=w322) -> ("AddressedToThisInstance?"=w320:bool)  [unwired: 8 in, 1 out]
            n283 = case shown="True" w320 {
              tunnel: [_ w325] -> w324
              tunnel: w323 -> [_ w329]
              frame False {
              }
              frame True {
                n284 = disable-structure shown="Enabled" {
                  disable-tunnel: "DeviceOff" ("Message") -> [w334 _]
                  disable-tunnel: w329 -> [w333 w335]
                  disable-tunnel: [w332 _] -> w328
                  disable-tunnel: [w331 w335] -> w327
                  frame Disabled {
                    n285 = call "Enqueue.vi"("Message"=w334, "MessageQueue"=w333) -> ("error out"=w332:errorcluster, "MessageQueue"=w331:refnum<queue>)  [unwired: 8 in]
                  }
                  frame Enabled {
                  }
                }
                n286 = call "Enqueue.vi"("error in (no error)"=w328, "Message"="Close", "MessageQueue"=w327) -> ("error out"=w325:errorcluster)  [unwired: 7 in, 1 out]
              }
            }
          }
        }
        n287 = call "ErrorHandler.vi"("error in (no error)"=w162, "MessageQueue"=w160) -> ("error out"=w161:errorcluster)  [unwired: 8 in, 1 out]
      }
    }
    frame Error {
      n288 = property class="ModuleAdmin.lvclass"(reference=w980) -> (reference out=w979:refnum<class "ModuleAdmin.lvclass">, "Accessors:CloneRegRef"=w978:refnum<data-value>, "Accessors:Module ID"=w977:i32)  [unwired: 1 in, 1 out]
      n289 = call <userlib>:"Remove.vi"("Module ID"=w977, "CloneRegRef"=w978) -> ("error out"=w981:errorcluster)  [unwired: 7 in, 2 out]
      n290 = flat-sequence {
        tunnel: w982 -> [w985]
        tunnel: w981 -> [_]
        tunnel: [w983] -> w972
        frame #0 {
          w984 = T6 2 items=["no dialog", "OK message", "continue or stop message", "OK message + warnings", "continue/stop + warnings"] ("type of dialog (OK msg:1)")
          n291 = call <vilib>:"Simple Error Handler.vi"("type of dialog (OK msg:1)"=w984, "error in (no error)"=w985) -> ("error out"=w983:errorcluster)  [unwired: 3 in, 4 out]
        }
      }
    }
  }
  n292 = call "DestroyClone.vi"("error in (no error)"=w3, "Exit via Stop Module Req?"=w41, "Wait for Module to stop?"=w42, "ModuleAdmin"=w4) -> ("error out"=w43:errorcluster, "External Launch"=w40:bool)  [unwired: 5 in, 1 out]
  n293 = Unregister For Events(event registration refnum=w38, error in=w39) -> (error out=w36:errorcluster)
  n294 = Release Queue(queue=w1, force destroy? (F)=w20, error in (no error)=w43) -> (error out=w28:errorcluster)  [unwired: 2 out]
  n295 = Release Queue(queue=w27, force destroy? (F)=w20, error in (no error)=w28) -> (error out=w19:errorcluster)  [unwired: 2 out]
  n296 = Release Queue(queue=w17, force destroy? (F)=w20, error in (no error)=w19) -> (error out=w18:errorcluster)  [unwired: 2 out]
  n297 = Merge Errors(w36, w18, w30) -> (w37:errorcluster)
  "error out" <- w37
  n298 = case shown="True" w40 {
    tunnel: w37 -> [_ w987]
    frame False {
    }
    frame True {
      n299 = control-ref of="This VI"() -> (w986:refnum<vi>)
      n300 = case shown="Error" w987 {
        tunnel: w986 -> [w989 w991]
        tunnel: [w988 w990] -> _
        frame No Error {
          n301 = invoke class="VI" method="FP.Close"(reference=w989) -> (error out=w988:errorcluster)  [unwired: 2 in, 2 out]
        }
        frame Error {
          n302 = invoke class="VI" method="FP.Open"(reference=w991, "Activate"=TRUE ("Activate?")) -> (error out=w990:errorcluster)  [unwired: 3 in, 4 out]
        }
      }
    }
  }
